vi "Polar Plot - Validate Rectangle.vi"(11 "rect":T1) -> (3 "valid rect":T1)   [LabVIEW 2020]
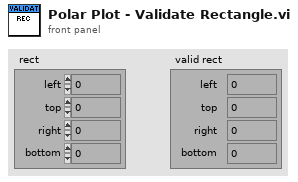
[diagram p1: front panel]
types:
  T1 = cluster{"left":i16, "top":i16, "right":i16, "bottom":i16}
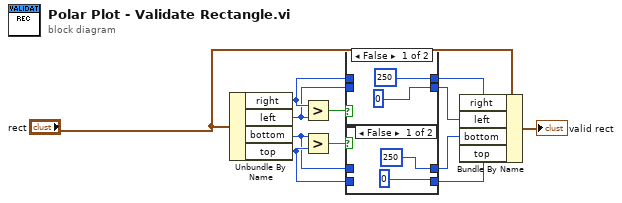
[diagram p0: block diagram]
diagram:
  n1 = Unbundle By Name("rect") -> ("right"=w11:i16, "left"=w10:i16, "bottom"=w7:i16, "top"=w8:i16)
  n2 = Greater?(x=w11, y=w10) -> (0:w12:bool)
  n3 = Greater?(x=w7, y=w8) -> (0:w9:bool)
  n4 = case shown="False" w12 {
    tunnel: w11 -> [_ w15]
    tunnel: w10 -> [_ w16]
    tunnel: [i16 0 w16] -> w3
    tunnel: [i16 250 w15] -> w6
    frame False {
    }
    frame True {
    }
  }
  n5 = case shown="False" w9 {
    tunnel: w8 -> [_ w20]
    tunnel: w7 -> [_ w19]
    tunnel: [i16 0 w20] -> w5
    tunnel: [i16 250 w19] -> w4
    frame False {
    }
    frame True {
    }
  }
  n6 = Bundle By Name(cluster="rect", "right"=w6, "left"=w3, "bottom"=w4, "top"=w5) -> (→"valid rect":T1)
